vi "SwerveModuleOdometry.vi"(4 "Robot Heading(deg)":dbl, 5 "Module Fault":bool, 7 "Wheel Azimuth (deg)":dbl, 9 "Velocity (ft/s)":dbl) -> (0 "Delta Y (in)":dbl, 1 "Delta X (in)":dbl, 2 "Velocity Y (ft/s)":dbl, 3 "Velocity X (ft/s)":dbl)   [LabVIEW 2020]
doc: "This VI calculates the field-centric delta odometry and velocity vectors for a single swerve module."
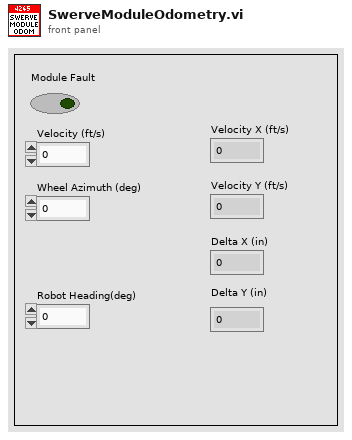
[diagram p1: front panel]
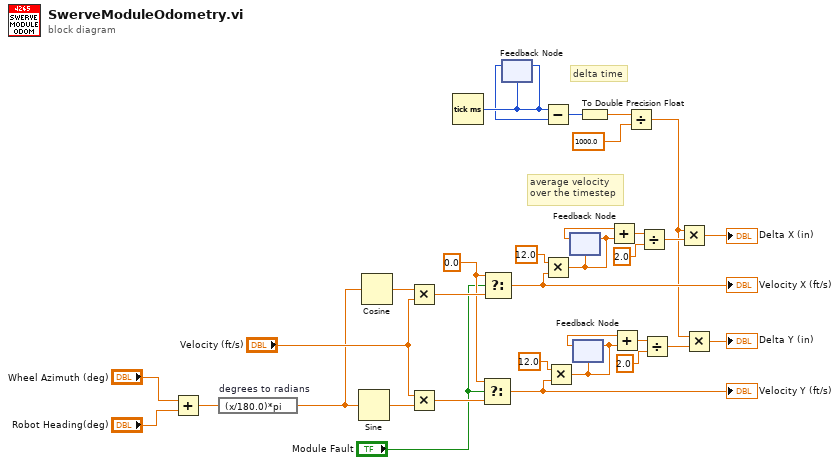
[diagram p0: block diagram]
diagram:
  w26 = 0.0 ("t")
  # "delta time"
  # "average velocity\nover the timestep"
  n1 = Add(x="Wheel Azimuth (deg)", y="Robot Heading(deg)") -> (x+y=w31:dbl)
  n2 = expression code="(x/180.0)*pi" "degrees to radians"(w31) -> (w19:dbl)
  n3 = Sine(x=w19) -> (sin(x)=w30:dbl)
  n4 = Cosine(x=w19) -> (cos(x)=w29:dbl)
  n5 = Multiply(x=w29, y="Velocity (ft/s)") -> (x*y=w28:dbl)
  n6 = Multiply(x="Velocity (ft/s)", y=w30) -> (x*y=w27:dbl)
  n7 = Tick Count (ms)() -> (millisecond timer value=w25:u32)
  n8 = Select(t=w26, s="Module Fault", f=w27) -> (s? t:f=w6:dbl)
  "Velocity Y (ft/s)" <- w6
  n9 = Select(t=w26, s="Module Fault", f=w28) -> (s? t:f=w16:dbl)
  "Velocity X (ft/s)" <- w16
  n10 = feedback-in #1(w25) -> ()
  n11 = feedback #1(w25) -> (w24:u32)
  n12 = Subtract(x=w25, y=w24) -> (x-y=w23:u32)
  n13 = Multiply(x=12.0 ("y"), y=w16) -> (x*y=w13:dbl)
  n14 = Multiply(x=12.0 ("y"), y=w6) -> (x*y=w8:dbl)
  n15 = feedback #2(w13) -> (w12:dbl)
  n16 = feedback-in #2(w13) -> ()
  n17 = feedback #3(w8) -> (w7:dbl)
  n18 = feedback-in #3(w8) -> ()
  n19 = To Double Precision Float(number=w23) -> (double precision float=w22:dbl)
  n20 = Add(x=w12, y=w13) -> (x+y=w15:dbl)
  n21 = Add(x=w7, y=w8) -> (x+y=w10:dbl)
  n22 = Divide(x=w22, y=1000.0) -> (x/y=w3:dbl)
  n23 = Divide(x=w15, y=2.0) -> (x/y=w5:dbl)
  n24 = Divide(x=w10, y=2.0) -> (x/y=w4:dbl)
  n25 = Multiply(x=w3, y=w5) -> (x*y=→"Delta X (in)":dbl)
  n26 = Multiply(x=w3, y=w4) -> (x*y=→"Delta Y (in)":dbl)
